vi "EventLogger.Manager.vi"(7 "action":T1=enum."get", 8 "error in":errorcluster, 11 "EventLog ref in":refnum<class "EventLog.lvclass">) -> (0 "error out":errorcluster, 3 "EventLog ref out":refnum<class "EventLog.lvclass">)   [LabVIEW 2019, in "Tools.lvlib"]
uses:
  Tools.lvlib
  EventLogger.Manager.Action.ctl
  <vilib>/NI/Event Logger Library/EventLog/EventLog.lvclass
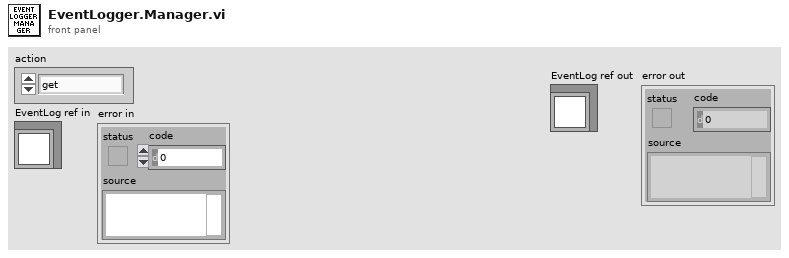
[diagram p1: front panel]
types:
  T1 = typedef "Tools.lvlib/EventLogger.Manager.Action.ctl" = enum16{"init", "get", "close"}
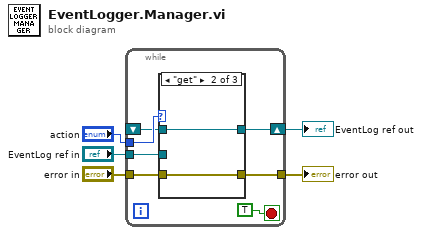
[diagram p0: block diagram]
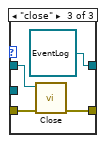
[diagram p3: hidden frame]
diagram:
  n1 = while {
    shift-right: [w10] -> w1
    shift-left: _ -> [w9]
    tunnel: "action" -> [w11]
    tunnel: "EventLog ref in" -> [w8]
    tunnel: "error in" -> [w7]
    tunnel: [w6] -> w2
    stop <- TRUE stop-if-true
    n2 = case shown="\"get\"" w11 {
      tunnel: [w14 w16 refnum<class "EventLog.lvclass"> refnum ("EventLog ref in")] -> w10
      tunnel: w9 -> [_ w16 w20]
      tunnel: w8 -> [w14 _ _]
      tunnel: w7 -> [w13 w15 w18]
      tunnel: [w13 w15 w17] -> w6
      frame "init" {
      }
      frame "get" {
      }
      frame "close" {
        n3 = call <vilib>:"Close.vi"("error in (no error)"=w18, "EventLog ref"=w20) -> ("error out"=w17:errorcluster)  [unwired: 9 in]
      }
    }
  }
  "EventLog ref out" <- w1
  "error out" <- w2
